vi "Write URI.vi"(8 "error in (no error)":errorcluster, 10 "URI":string, 11 "ConfigManager in":refnum<class "ConfigManager.lvclass">) -> (0 "error out":errorcluster, 3 "ConfigManager out":refnum<class "ConfigManager.lvclass">)   [LabVIEW 2013, in "CfgManager.lvlib" / "ConfigManager.lvclass"]
uses:
  ConfigManager.lvclass
  ConfigManager.lvclass/ConfigManager.ctl
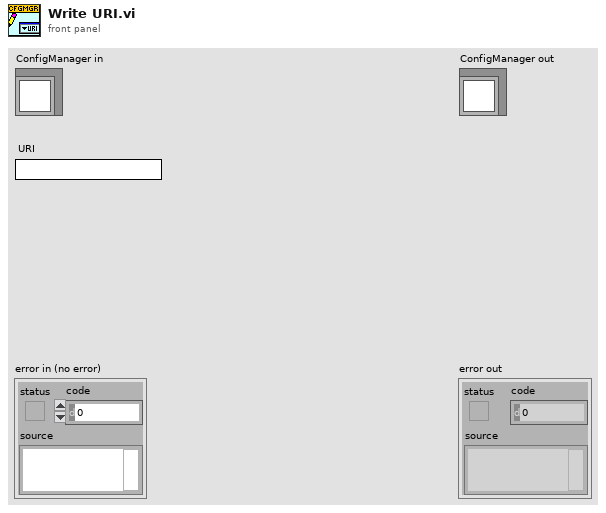
[diagram p1: front panel]
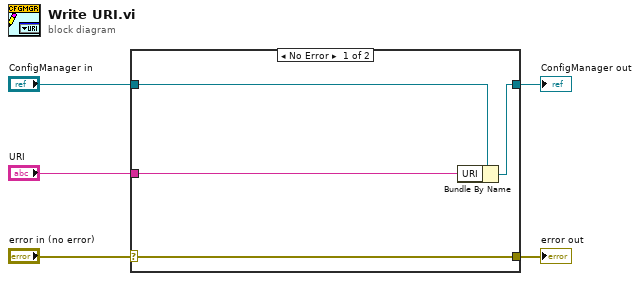
[diagram p0: block diagram]
diagram:
  n1 = case shown="No Error" "error in (no error)" {
    selector: "error in (no error)" -> [w9 w10]
    tunnel: [w9 w10] -> w4
    tunnel: [w7 w11] -> w2
    tunnel: "ConfigManager in" -> [w8 w11]
    tunnel: "URI" -> [w6 _]
    frame No Error {
      n2 = Bundle By Name(cluster=w8, "URI"=w6) -> (w7:refnum<class "ConfigManager.lvclass">)
    }
    frame Error {
    }
  }
  "error out" <- w4
  "ConfigManager out" <- w2
